vi "set_resolution.vi"(7 "get from XImage (F)":bool, 8 "error in (no error)":errorcluster, 9 "y resolution":u32, 10 "x resolution":u32, 11 "TrajectoryMH100122AODRAPS in":refnum<class "TrajectoryMH100122AODRAPS.lvclass">) -> (0 "error out":errorcluster, 3 "TrajectoryMH100122AODRAPS out":refnum<class "TrajectoryMH100122AODRAPS.lvclass">)   [LabVIEW 2010, in "TrajectoryMH100122AODRAPS.lvclass"]
uses:
  TrajectoryMH100122AODRAPS.lvclass
  common/xcontrols/XImage/XImage/XImage.xctl
  TrajectoryMH100122AODRAPS.lvclass/TrajectoryMH100122AODRAPS.ctl
  class_data.vi
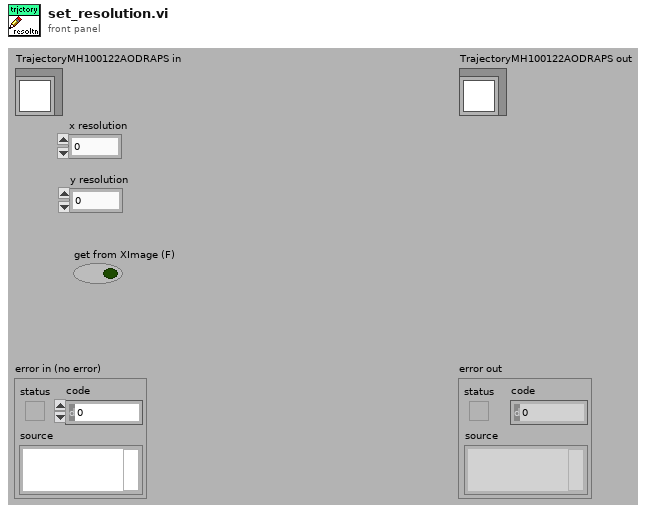
[diagram p1: front panel]
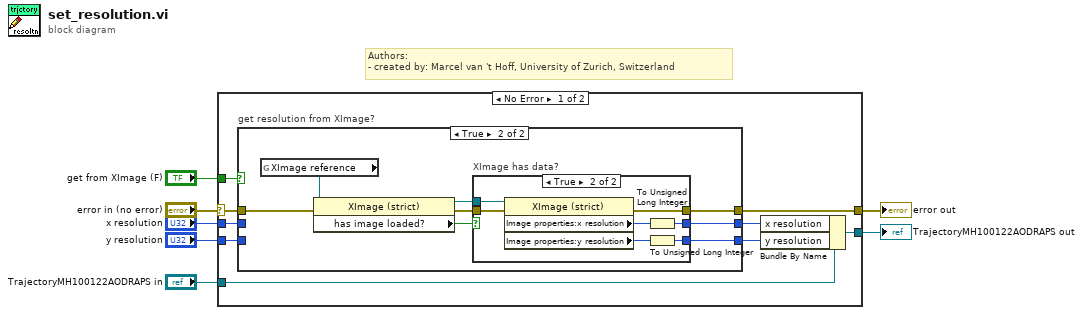
[diagram p0: block diagram]
diagram:
  # "Authors: \n- created by: Marcel van 't Hoff, University of Zurich, Switzerland"
  n1 = case shown="No Error" "error in (no error)" {
    selector: "error in (no error)" -> [w9 w37]
    tunnel: [w8 w37] -> w6
    tunnel: [w15 w36] -> w4
    tunnel: "TrajectoryMH100122AODRAPS in" -> [w16 w36]
    tunnel: "get from XImage (F)" -> [w14 _]
    tunnel: "y resolution" -> [w13 _]
    tunnel: "x resolution" -> [w12 _]
    frame No Error {
      n2 = case "get resolution from XImage?" shown="True" w14 {
        tunnel: w13 -> [w18 _]
        tunnel: w12 -> [w19 _]
        tunnel: [w19 w27] -> w11
        tunnel: [w18 w26] -> w10
        tunnel: w9 -> [w17 w24]
        tunnel: [w17 w25] -> w8
        frame False {
        }
        frame True {
          n3 = global read "class_data.vi" "XImage reference"() -> (w22:refnum<vi>)
          n4 = property class="XImage (strict)"(reference=w22, error in=w24) -> (reference out=w21:refnum<vi>, error out=w23:errorcluster, "has image loaded?"=w20:bool)
          n5 = case "XImage has data?" shown="True" w20 {
            tunnel: [_ w33] -> w27
            tunnel: [_ w32] -> w26
            tunnel: w23 -> [w28 w31]
            tunnel: [w28 w30] -> w25
            tunnel: w21 -> [_ w29]
            frame False {
            }
            frame True {
              n6 = property class="XImage (strict)"(reference=w29, error in=w31) -> (error out=w30:errorcluster, "Image properties:x resolution"=w35:i32, "Image properties:y resolution"=w34:i32)  [unwired: 1 out]
              n7 = To Unsigned Long Integer(number=w35) -> (unsigned 32bit integer=w33:u32)
              n8 = To Unsigned Long Integer(number=w34) -> (unsigned 32bit integer=w32:u32)
            }
          }
        }
      }
      n9 = Bundle By Name(cluster=w16, "x resolution"=w11, "y resolution"=w10) -> (w15:refnum<class "TrajectoryMH100122AODRAPS.lvclass">)
    }
    frame Error {
    }
  }
  "error out" <- w6
  "TrajectoryMH100122AODRAPS out" <- w4
